vi "ep_Simulate Calibration Instrument.vi"(0 "frequency [Hz]":dbl=50.0, 1 "output state (F: OFF)":bool, 2 "harmonics state (F: OFF)":bool, 5 "voltage RMS [V]":dbl=230.0, 7 "current RMS [A]":dbl=1.0, 9 "harmonics":T1={"harmonic"=3, "voltage amplitude [%]"=10.0, "voltage phase [°]"=0.0, "current amplitude [%]"=10.0, "current phase [°]"=0.0}) -> (4 "Instrument voltage signal output":dbl[](graph), 6 "Instrument current signal output":dbl[](graph))   [LabVIEW 2012]
uses:
  <vilib>/Analysis/NI_AALBase.lvlib
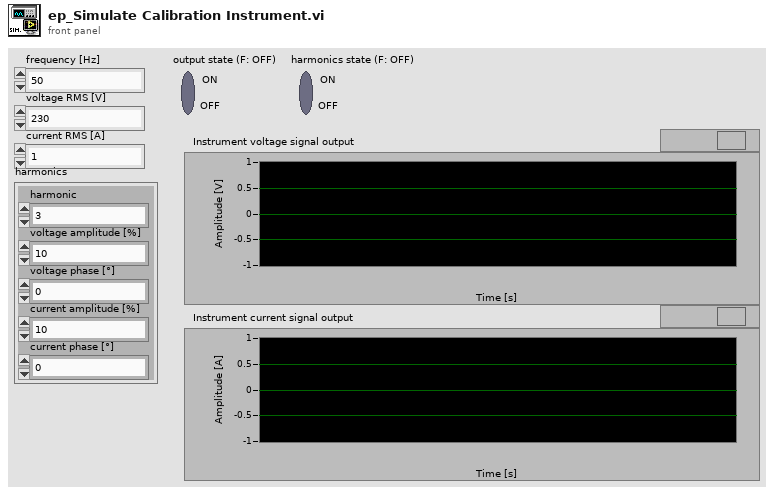
[diagram p1: front panel]
types:
  T1 = cluster{"harmonic":u32, "voltage amplitude [%]":dbl, "voltage phase [°]":dbl, "current amplitude [%]":dbl, "current phase [°]":dbl}
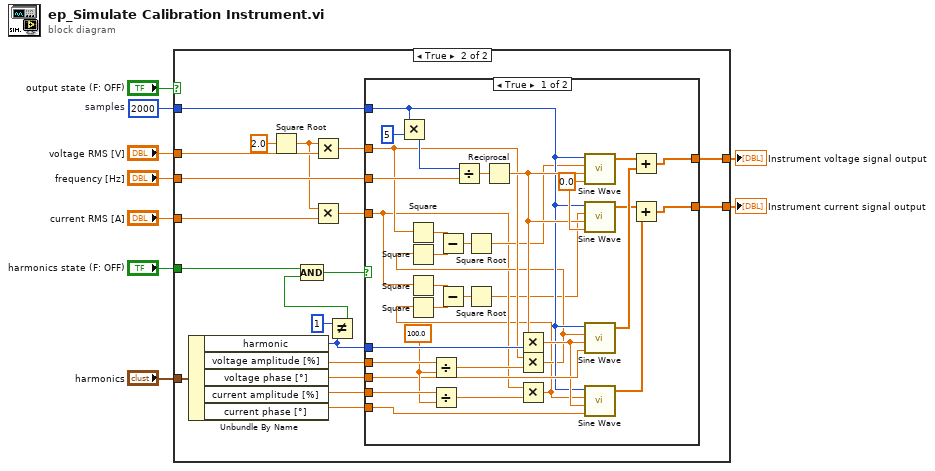
[diagram p0: block diagram]
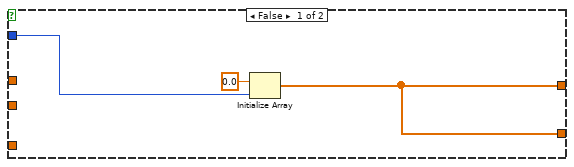
[diagram p2: hidden frame]
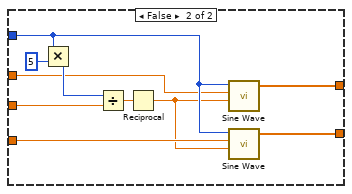
[diagram p3: hidden frame]
diagram:
  w6 = 2000  # samples
  n1 = case shown="True" "output state (F: OFF)" {
    tunnel: "voltage RMS [V]" -> [_ w17]
    tunnel: [w10 w32] -> w2
    tunnel: "frequency [Hz]" -> [_ w31]
    tunnel: w6 -> [w12 w30]
    tunnel: "harmonics" -> [_ w29]
    tunnel: "harmonics state (F: OFF)" -> [_ w27]
    tunnel: "current RMS [A]" -> [_ w15]
    tunnel: [w10 w24] -> w1
    frame False {
      n2 = Initialize Array(0.0, w12) -> (w10:dbl[])
    }
    frame True {
      n3 = Unbundle By Name(w29) -> ("harmonic"=w23:u32, "voltage amplitude [%]"=w22:dbl, "voltage phase [°]"=w20:dbl, "current amplitude [%]"=w21:dbl, "current phase [°]"=w19:dbl)
      n4 = Square Root(x=2.0) -> (sqrt(x)=w13:dbl)
      n5 = Multiply(x=w13, y=w17) -> (x*y=w16:dbl)
      n6 = Multiply(x=w13, y=w15) -> (x*y=w14:dbl)
      n7 = Not Equal?(x=u32 1, y=w23) -> (x != y?=w26:bool)
      n8 = Compound Arithmetic op=AND(w27, w26) -> (w25:bool)
      n9 = case shown="True" w25 {
        tunnel: [w53 w76] -> w32
        tunnel: w31 -> [w65 w74]
        tunnel: w30 -> [w50 w71]
        tunnel: w16 -> [w44 w70]
        tunnel: w14 -> [w35 w69]
        tunnel: [w46 w68] -> w24
        tunnel: w23 -> [w62 _]
        tunnel: w22 -> [w61 _]
        tunnel: w21 -> [w58 _]
        tunnel: w20 -> [w56 _]
        tunnel: w19 -> [w49 _]
        frame True {
          w59 = 0.0 ("phase in")
          w57 = 100.0 ("y")
          n10 = Multiply(x=w50, y=5) -> (x*y=w63:i32)
          n11 = Square(x=w44) -> (x^2=w42:dbl)
          n12 = Square(x=w35) -> (x^2=w36:dbl)
          n13 = Divide(x=w61, y=w57) -> (x/y=w60:dbl)
          n14 = Divide(x=w58, y=w57) -> (x/y=w45:dbl)
          n15 = Divide(x=w63, y=w65) -> (x/y=w66:dbl)
          n16 = Reciprocal(x=w66) -> (1/x=w52:dbl)
          n17 = Multiply(x=w52, y=w62) -> (x*y=w51:dbl)
          n18 = Multiply(x=w44, y=w60) -> (x*y=w43:dbl)
          n19 = Square(x=w43) -> (x^2=w41:dbl)
          n20 = Subtract(x=w42, y=w41) -> (x-y=w40:dbl)
          n21 = Square Root(x=w40) -> (sqrt(x)=w39:dbl)
          n22 = Multiply(x=w35, y=w45) -> (x*y=w34:dbl)
          n23 = Square(x=w34) -> (x^2=w37:dbl)
          n24 = Subtract(x=w36, y=w37) -> (x-y=w38:dbl)
          n25 = Square Root(x=w38) -> (sqrt(x)=w33:dbl)
          n26 = call <vilib>:"Sine Wave.vi"("samples"=w50, "amplitude"=w39, "frequency"=w52, "phase in"=w59) -> ("sine wave"=w54:dbl[])  [unwired: 1 in, 2 out]
          n27 = call <vilib>:"Sine Wave.vi"("samples"=w50, "amplitude"=w33, "frequency"=w52, "phase in"=w59) -> ("sine wave"=w47:dbl[])  [unwired: 1 in, 2 out]
          n28 = call <vilib>:"Sine Wave.vi"("samples"=w50, "amplitude"=w43, "frequency"=w51, "phase in"=w56) -> ("sine wave"=w55:dbl[])  [unwired: 1 in, 2 out]
          n29 = call <vilib>:"Sine Wave.vi"("samples"=w50, "amplitude"=w34, "frequency"=w51, "phase in"=w49) -> ("sine wave"=w48:dbl[])  [unwired: 1 in, 2 out]
          n30 = Add(x=w54, y=w55) -> (x+y=w53:dbl[])
          n31 = Add(x=w47, y=w48) -> (x+y=w46:dbl[])
        }
        frame False {
          n32 = Multiply(x=w71, y=5) -> (x*y=w72:i32)
          n33 = Divide(x=w72, y=w74) -> (x/y=w75:dbl)
          n34 = Reciprocal(x=w75) -> (1/x=w67:dbl)
          n35 = call <vilib>:"Sine Wave.vi"("samples"=w71, "amplitude"=w70, "frequency"=w67) -> ("sine wave"=w76:dbl[])  [unwired: 2 in, 2 out]
          n36 = call <vilib>:"Sine Wave.vi"("samples"=w71, "amplitude"=w69, "frequency"=w67) -> ("sine wave"=w68:dbl[])  [unwired: 2 in, 2 out]
        }
      }
    }
  }
  "Instrument current signal output" <- w1
  "Instrument voltage signal output" <- w2
